vi "Untitled 2 (SubVI).vi"(11 "Numeric":dbl) -> (3 "number (0 to 1)":dbl)   [LabVIEW 2015]
panel:
  in  "number (0 to 1) 2":dbl
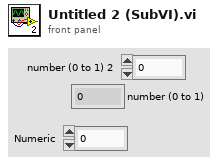
[diagram p1: front panel]
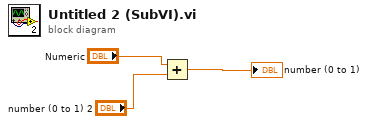
[diagram p0: block diagram]
diagram:
  n1 = Add(x="Numeric", y="number (0 to 1) 2") -> (x+y=→"number (0 to 1)":dbl)
